vi "Create Test Configuration.vi"() -> (0 "error out":errorcluster, 1 "Names":string[](array[string]), 2 "Line Array":T1[](array[typedef]), 3 "Module Configuration":refnum<class "Missing Plugin configuration.lvclass">, 4 "Channels":refnum<class "TBM channel.lvclass">[](array[class]), 5 "instance identifier":string)   [LabVIEW 2014, in "Missing Plugin tests.lvlib"]
doc: "This VI creates a standard test configuration for other unit tests. It currently creates and adds one line with every datatype to the module configuration."
uses:
  Missing Plugin tests.lvlib
  module/configuration/Missing Plugin configuration.lvclass
  module/configuration/Line.ctl
  <vilib>/NI/Tag Bus Module Framework/channel/TBM channel.lvclass
  <vilib>/NI/Tag Bus Module Framework/channel/channel classification.ctl
  <vilib>/NI/Configuration Framework/serializable configuration/NISE_CEF_serializable configuration.lvclass
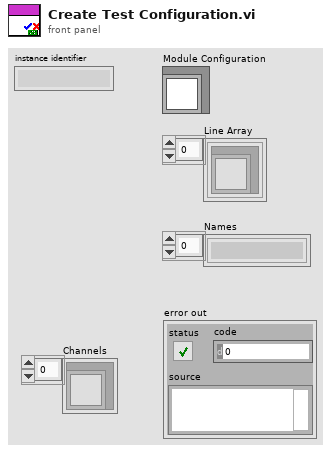
[diagram p1: front panel]
types:
  T1 = typedef "Missing Plugin configuration.lvclass/Line.ctl" = cluster{"channel":refnum<class "TBM channel.lvclass">}
  T2 = typedef "TBM channel.lvclass/channel classification.ctl" = enum16{"input data", "output data", "processing parameter", "processing result"}
  T3 = typedef "tag bus.lvlib/tag descriptor.lvclass/Data Type.ctl" = enum16{"Double", "Single", "I64", "I32", "I16", "I8", "U64", "U32", "U16", "U8", "Boolean", "String", "Array of Double", "Array of Single", "Array of I64", "Array of I32", "Array of I16", "Array of I8", "Array of U64", "Array of U32", "Array of U16", "Array of U8", "Array of Boolean", "Array of String"}
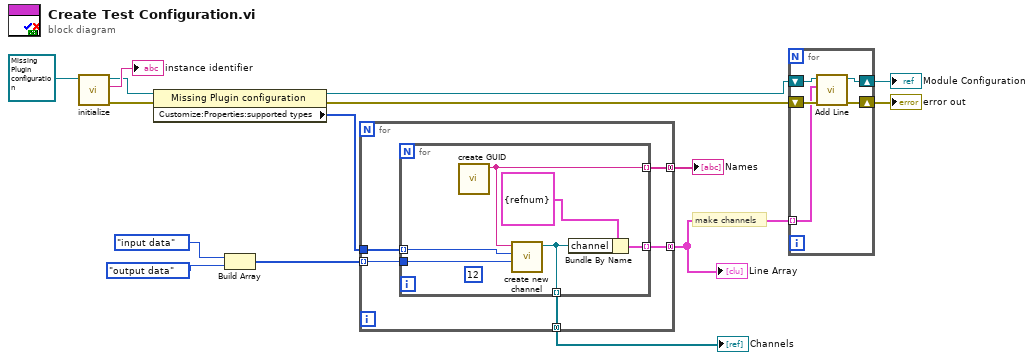
[diagram p0: block diagram]
diagram:
  # "make channels"
  n1 = call <vilib>:"initialize.vi"("configuration in"=refnum<class "Missing Plugin configuration.lvclass"> refnum ("tag bus configurable plugin module configuration")) -> ("error out"=w13:errorcluster, "identifier"=→"instance identifier":string, "configuration out"=w10:refnum<class "Missing Plugin configuration.lvclass">)  [unwired: 8 in]
  n2 = property class="Missing Plugin configuration"(reference=w10, error in=w13) -> (reference out=w5:refnum<class "Missing Plugin configuration.lvclass">, error out=w12:errorcluster, "Customize:Properties:supported types"=w6:T3[])
  n3 = Build Array(channel_classification."input data" ("channel classification"), channel_classification."output data" ("channel classification")) -> (w4:T2[])
  n4 = for {
    tunnel: w4 -> [w20] mode=indexing
    tunnel: [w18] -> w9 mode=concatenating
    tunnel: w6 -> [w19]
    tunnel: [w17] -> w11 mode=concatenating
    tunnel: [w16] -> w1 mode=concatenating
    n5 = for {
      tunnel: w20 -> [w26]
      tunnel: [w22] -> w18 mode=indexing
      tunnel: w19 -> [w25] mode=indexing
      tunnel: [w24] -> w17 mode=indexing
      tunnel: [w21] -> w16 mode=indexing
      (unwired) 12
      n6 = call <vilib>:"create GUID.vi"() -> ("uuid"=w24:string)  [unwired: 10 in, 1 out]
      n7 = call <vilib>:"create new channel.vi"("channel classification"=w26, "data type"=w25, "channel name"=w24) -> ("channel"=w21:refnum<class "TBM channel.lvclass">)  [unwired: 8 in]
      n8 = Bundle By Name(cluster=T1 {"channel"=refnum} ("Line"), "channel"=w21) -> (w22:T1)
    }
  }
  "Names" <- w11
  "Line Array" <- w9
  "Channels" <- w1
  n9 = for {
    tunnel: w9 -> [w27] mode=indexing
    shift-right: [w30] -> w8
    shift-left: w5 -> [w31]
    shift-right: [w28] -> w15
    shift-left: w12 -> [w29]
    n10 = call "Add Line.vi"("error in"=w29, "Line"=w27, "Missing Plugin configuration in"=w31) -> ("error out"=w28:errorcluster, "Missing Plugin configuration out"=w30:refnum<class "Missing Plugin configuration.lvclass">)  [unwired: 6 in, 1 out]
  }
  "error out" <- w15
  "Module Configuration" <- w8
